vi "Counter.vi"(0 "Pulse/Trig Cluster":T1={"Digital Trigger Source"="/6602/PFI39", "Edge"=10280, "Number of Pulses"=1000, "High time"=1e-07, "Low time"=2e-07, "Output Terminal"="/6602/PXI_Trig0", "Counter"="6602/ctr0"} {"Low time" format="%.0p"; "High time" format="%.0p"; "Edge" items=["Rising"=10280, "Falling"=10171]}) -> (1 "task out":refnum<k21>, 2 "error out":errorcluster)   [LabVIEW 2018]
doc: "This example demonstrates how to generate a finite number of digital pulses using a counter output.\n\nOn some hardware, this requires the use of a second counter to generate a gate signal. If necessary, DAQmx configures this second counter for you."
uses:
  <vilib>/Utility/error.llb/DialogType.ctl
  <vilib>/DAQmx/create/channels.llb/DAQmx Create Channel (CO-Pulse Generation-Time).vi
  <vilib>/DAQmx/configure/timing.llb/DAQmx Timing (Implicit).vi
  <vilib>/DAQmx/configure/trigger.llb/DAQmx Start Trigger (Digital Edge).vi
  <resource>/objmgr/daqmx.rc
panel:
  in  "Wait1 (us)":u32=8000
  out "t3":u32=11204
  in  "Number of Pulses 2":i32=1000
  in  "Wait2 (uSec)":u32=5000 caption="Wait2 (us)"
  out "t4":u32=17006
  out "t2":u32=10015
  out "t1":u32=2000
  out "microsecond timer value":u32=2969608980
  in  "Number of Pulses":i32=1000
  in  "Low time":dbl=2e-07 format="%.0p"
  in  "High time":dbl=1e-07 format="%.0p"
  in  "Output Terminal":tag="/6602/PXI_Trig0"
  in  "Trigger Type":enum32{"No Trigger", "Digital Start"}(tab)
  in  "Retriggerable":bool
  in  "Edge":i32(ring)=10280 items=["Rising"=10280, "Falling"=10171]
  in  "Digital Trigger Source":tag="/6602/PFI39"
  in  "Stop":bool
  in  "Counter":tag="6602/ctr0"
  # "Channel Settings"
  # "Timing Settings"
  # "Trigger Settings"
  # "6602 can have much shorter Wait2\nthan 6723 or 6733, independent of trig source, output term"
  # "To configure and use a trigger you must have the necessary tab selected above."
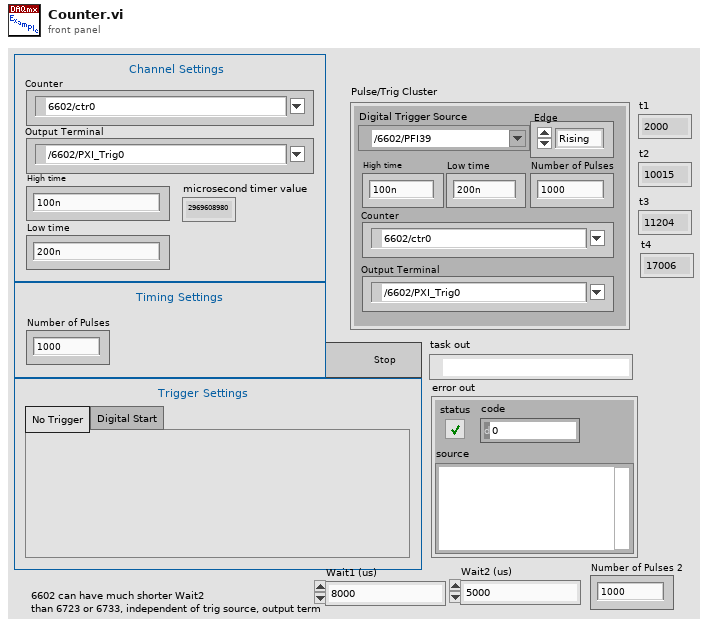
[diagram p1: front panel]
types:
  T1 = cluster{"Digital Trigger Source":tag, "Edge":i32, "Number of Pulses":i32, "High time":dbl, "Low time":dbl, "Output Terminal":tag, "Counter":tag}
  T2 = typedef "DialogType.ctl" = u16
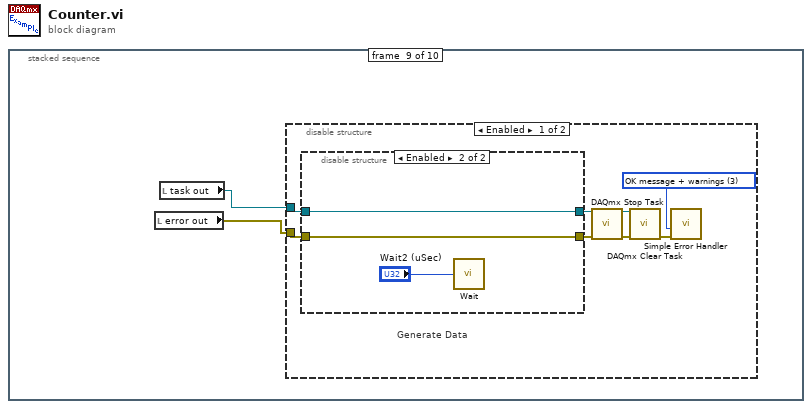
[diagram p0: block diagram]
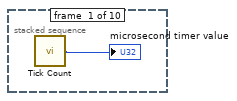
[diagram p2: hidden frame]
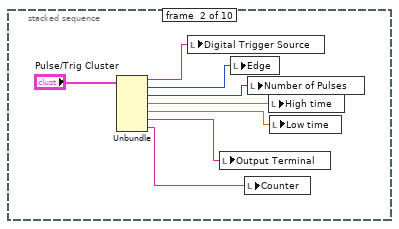
[diagram p3: hidden frame]
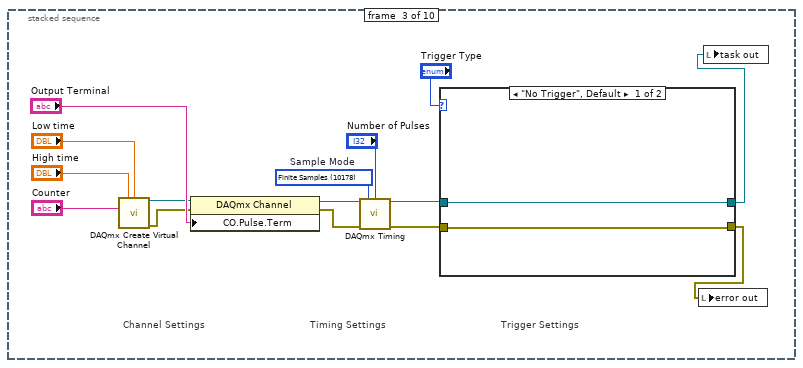
[diagram p4: hidden frame]
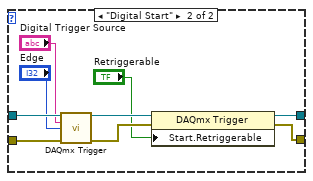
[diagram p5: hidden frame]
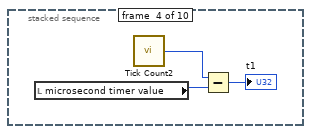
[diagram p6: hidden frame]
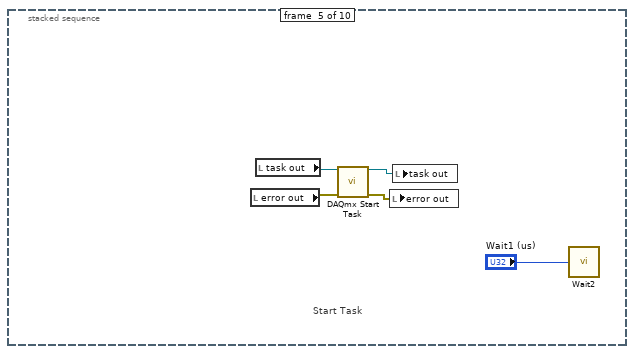
[diagram p7: hidden frame]
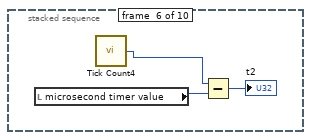
[diagram p8: hidden frame]
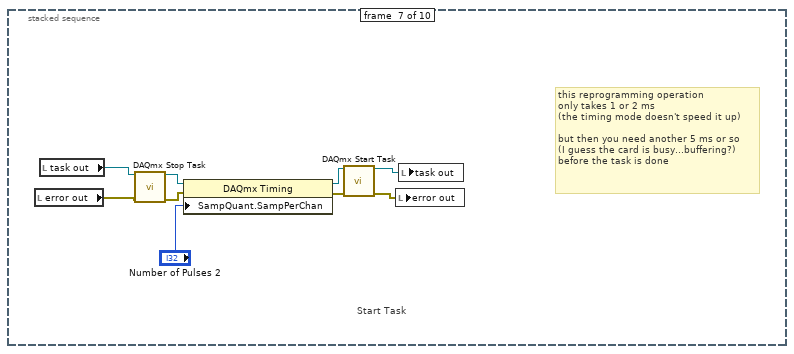
[diagram p9: hidden frame]
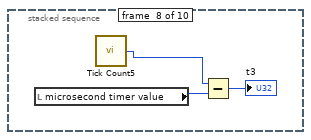
[diagram p10: hidden frame]
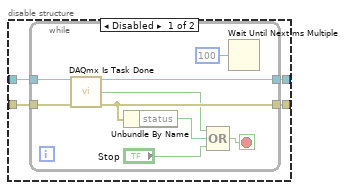
[diagram p11: hidden frame]
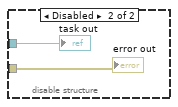
[diagram p12: hidden frame]
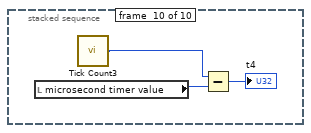
[diagram p13: hidden frame]
diagram:
  n1 = stacked-sequence {
    frame #0 {
      n2 = call "Tick Count"() -> ("Tick Count(uSec)"=→"microsecond timer value":u32)
    }
    frame #1 {
      n3 = Unbundle("Pulse/Trig Cluster") -> ("Digital Trigger Source"=w7:tag, "Edge"=w8:i32, "Number of Pulses"=w6:i32, "High time"=w5:dbl, "Low time"=w4:dbl, "Output Terminal"=w3:tag, "Counter"=w2:tag)
      n4 = local write "Digital Trigger Source"(w7) -> ()
      n5 = local write "Output Terminal"(w3) -> ()
      n6 = local write "Edge"(w8) -> ()
      n7 = local write "Counter"(w2) -> ()
      n8 = local write "Number of Pulses"(w6) -> ()
      n9 = local write "High time"(w5) -> ()
      n10 = local write "Low time"(w4) -> ()
    }
    frame #2 {
      w12 = 10178 items=["Finite Samples"=10178, "Continuous Samples"=10123, "Hardware Timed Single Point"=12522]  # Sample Mode
      # "Trigger Settings"
      # "Timing Settings"
      # "Channel Settings"
      n11 = call-poly <vilib>:"DAQmx Create Virtual Channel.vi"("high time"="High time", "low time"="Low time", "counter"="Counter") -> ("task out"=w17:refnum<k21>, "error out"=w18:errorcluster)  [unwired: 11 in]
      n12 = property class="DAQmx Channel"(reference=w17, error in=w18, "CO.Pulse.Term"="Output Terminal") -> (reference out=w21:refnum<k21>, error out=w20:errorcluster)
      n13 = call-poly <vilib>:"DAQmx Timing.vi"("task/channels in"=w21, "sample mode"=w12, "samples per channel"="Number of Pulses", "error in"=w20) -> ("task out"=w15:refnum<k21>, "error out"=w16:errorcluster)  [unwired: 10 in]
      n14 = case shown="\"No Trigger\", Default" "Trigger Type" {
        tunnel: w15 -> [w26 w35]
        tunnel: w16 -> [w25 w34]
        tunnel: [w26 w31] -> w10
        tunnel: [w25 w30] -> w11
        frame "No Trigger", Default {
        }
        frame "Digital Start" {
          n15 = call-poly <vilib>:"DAQmx Trigger.vi"("task/channels in"=w35, "source"="Digital Trigger Source", "edge"="Edge", "error in"=w34) -> ("task out"=w28:refnum<k21>, "error out"=w29:errorcluster)  [unwired: 10 in]
          n16 = property class="DAQmx Trigger"(reference=w28, error in=w29, "Start.Retriggerable"="Retriggerable") -> (reference out=w31:refnum<k21>, error out=w30:errorcluster)
        }
      }
      n17 = local write "error out"(w11) -> ()
      n18 = local write "task out"(w10) -> ()
    }
    frame #3 {
      n19 = local read "microsecond timer value"() -> (w38:u32)
      n20 = call "Tick Count2"() -> ("Tick Count(uSec)"=w37:u32)
      n21 = Subtract(x=w37, y=w38) -> (x-y=→"t1":u32)
    }
    frame #4 {
      # "Start Task"
      n22 = local read "error out"() -> (w42:errorcluster)
      n23 = local read "task out"() -> (w43:refnum<k21>)
      n24 = call <vilib>:"DAQmx Start Task.vi"("task/channels in"=w43, "error in"=w42) -> ("task out"=w40:refnum<k21>, "error out"=w41:errorcluster)  [unwired: 12 in]
      n25 = local write "error out"(w41) -> ()
      n26 = local write "task out"(w40) -> ()
      n27 = call "Wait2"("Count(uSec)"="Wait1 (us)") -> ()  [unwired: 1 out]
    }
    frame #5 {
      n28 = local read "microsecond timer value"() -> (w46:u32)
      n29 = call "Tick Count4"() -> ("Tick Count(uSec)"=w44:u32)
      n30 = Subtract(x=w44, y=w46) -> (x-y=→"t2":u32)
    }
    frame #6 {
      # "this reprogramming operation\nonly takes 1 or 2 ms\n(the timing mode doesn't speed it up)\n\nbut then you need another 5 ms or so\n(I guess the card is busy...buffering?)\nbefore the task is done"
      # "Start Task"
      n31 = local read "error out"() -> (w53:errorcluster)
      n32 = local read "task out"() -> (w52:refnum<k21>)
      n33 = call <vilib>:"DAQmx Stop Task.vi"("task/channels in"=w52, "error in"=w53) -> ("task out"=w51:refnum<k21>, "error out"=w50:errorcluster)  [unwired: 12 in]
      n34 = property class="DAQmx Timing"(reference=w51, error in=w50, "SampQuant.SampPerChan"="Number of Pulses 2") -> (reference out=w49:refnum<k21>, error out=w48:errorcluster)
      n35 = call <vilib>:"DAQmx Start Task.vi"("task/channels in"=w49, "error in"=w48) -> ("task out"=w54:refnum<k21>, "error out"=w55:errorcluster)  [unwired: 12 in]
      n36 = local write "error out"(w55) -> ()
      n37 = local write "task out"(w54) -> ()
    }
    frame #7 {
      n38 = local read "microsecond timer value"() -> (w58:u32)
      n39 = call "Tick Count5"() -> ("Tick Count(uSec)"=w56:u32)
      n40 = Subtract(x=w56, y=w58) -> (x-y=→"t3":u32)
    }
    frame #8 {
      n41 = local read "error out"() -> (w59:errorcluster)
      n42 = local read "task out"() -> (w60:refnum<k21>)
      n43 = disable-structure shown="Enabled" {
        disable-tunnel: w60 -> [w68 w86]
        disable-tunnel: w59 -> [w67 w85]
        frame Enabled {
          w61 = T2 3 items=["no dialog", "OK message", "continue or stop message", "OK message + warnings", "continue/stop + warnings"] ("type of dialog (OK msg:1)")
          # "Generate Data"
          n44 = disable-structure shown="Enabled" {
            disable-tunnel: w68 -> [w72 w84]
            disable-tunnel: w67 -> [w71 w83]
            disable-tunnel: [w70 w84] -> w63
            disable-tunnel: [w69 w83] -> w62
            frame Disabled {
              n45 = while {
                tunnel: w72 -> [w81]
                tunnel: w71 -> [w80]
                tunnel: [w77] -> w69
                tunnel: [w78] -> w70
                stop <- w79 stop-if-true
                n46 = call <vilib>:"DAQmx Is Task Done.vi"("task/channels in"=w81, "error in"=w80) -> ("task out"=w78:refnum<k21>, "task done?"=w73:bool, "error out"=w77:errorcluster)  [unwired: 11 in]
                n47 = Unbundle By Name(w77) -> ("status"=w76:bool)
                n48 = Compound Arithmetic op=OR(w73, w76, "Stop") -> (w79:bool)
                n49 = Wait Until Next ms Multiple(millisecond multiple=u32 100) -> ()  [unwired: 1 out]
              }
            }
            frame Enabled {
              n50 = call "Wait"("Count(uSec)"="Wait2 (uSec)") -> ()  [unwired: 1 out]
            }
          }
          n51 = call <vilib>:"DAQmx Stop Task.vi"("task/channels in"=w63, "error in"=w62) -> ("task out"=w65:refnum<k21>, "error out"=w64:errorcluster)  [unwired: 12 in]
          n52 = call <vilib>:"DAQmx Clear Task.vi"("task in"=w65, "error in"=w64) -> ("error out"=w66:errorcluster)  [unwired: 13 in]
          n53 = call <vilib>:"Simple Error Handler.vi"("type of dialog (OK msg:1)"=w61, "error in (no error)"=w66) -> ()  [unwired: 3 in, 5 out]
        }
        frame Disabled {
          "task out" <- w86
          "error out" <- w85
        }
      }
    }
    frame #9 {
      n54 = local read "microsecond timer value"() -> (w89:u32)
      n55 = call "Tick Count3"() -> ("Tick Count(uSec)"=w87:u32)
      n56 = Subtract(x=w87, y=w89) -> (x-y=→"t4":u32)
    }
  }
